vi "harp_connection_save_to_dev.vi"(0 "port in":refnum<visa-resource-name>) -> (4 "port out":refnum<visa-resource-name>, 8 "port closed":bool caption="Boolean", 15 "error out":errorcluster)   [LabVIEW 2010]
panel:
  in  "Visual Indicators:":enum8{"ON", "OFF"}(ring)
  in  "reset":bool caption="Boolean"
  in  "cancel":bool caption="Boolean"
  in  "LED State:":enum8{"ON", "OFF"}(ring)
  in  "Device State:":enum8{"Standby", "Active"}(ring)
  in  "read 5":bool
  in  "read 4":bool
  in  "read":bool
  in  "read 6":bool
  in  "read 7":bool
  in  "read 8":bool
  in  "read 3":bool
  in  "device":refnum<visa-resource-name>="COM5"
  in  "OK":bool caption="Boolean"
  # "Define the default state off the device."
  # "Configuration:"
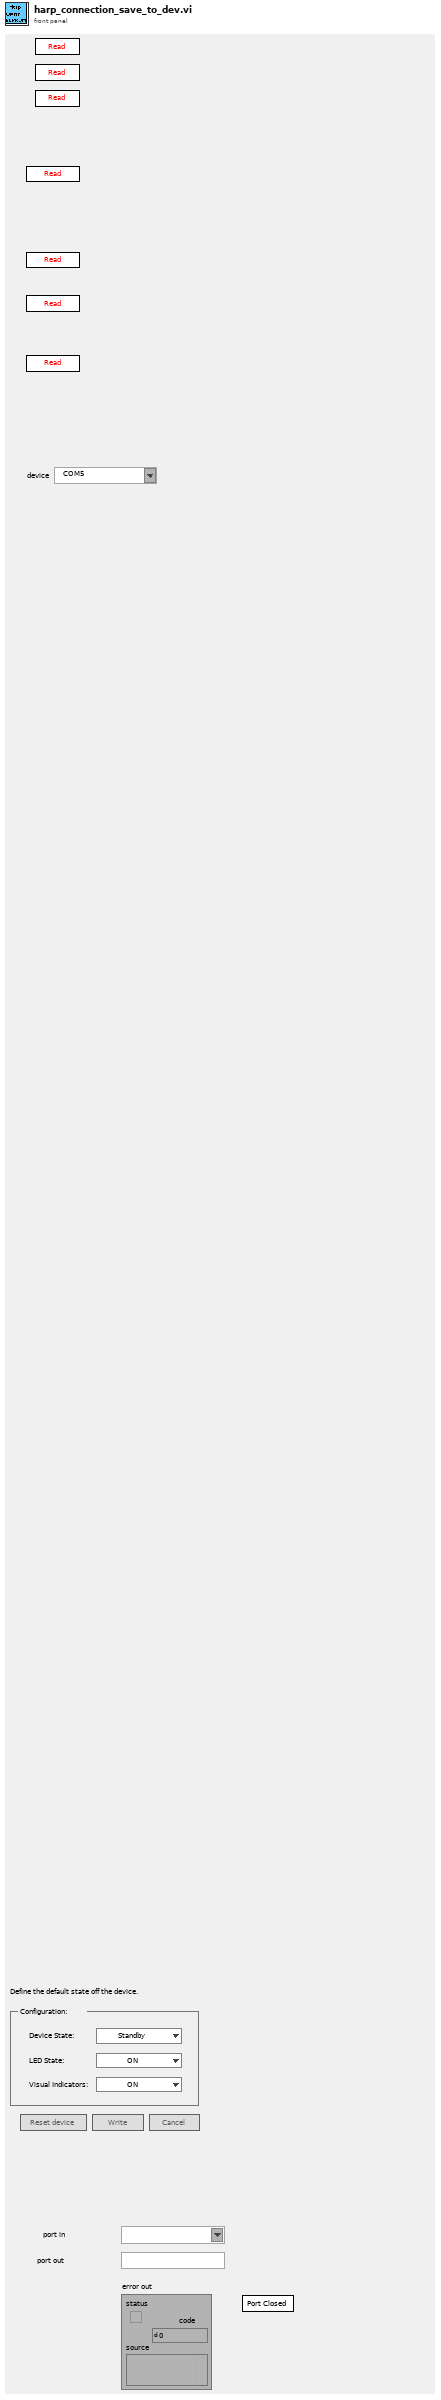
[diagram p1: front panel]
types:
  T1 = enum8{"Enabled", "Disabled", "Disabled and Grayed Out"}
  T2 = enum16{"Left Button", "Center Button", "Right Button", "Window Close"}
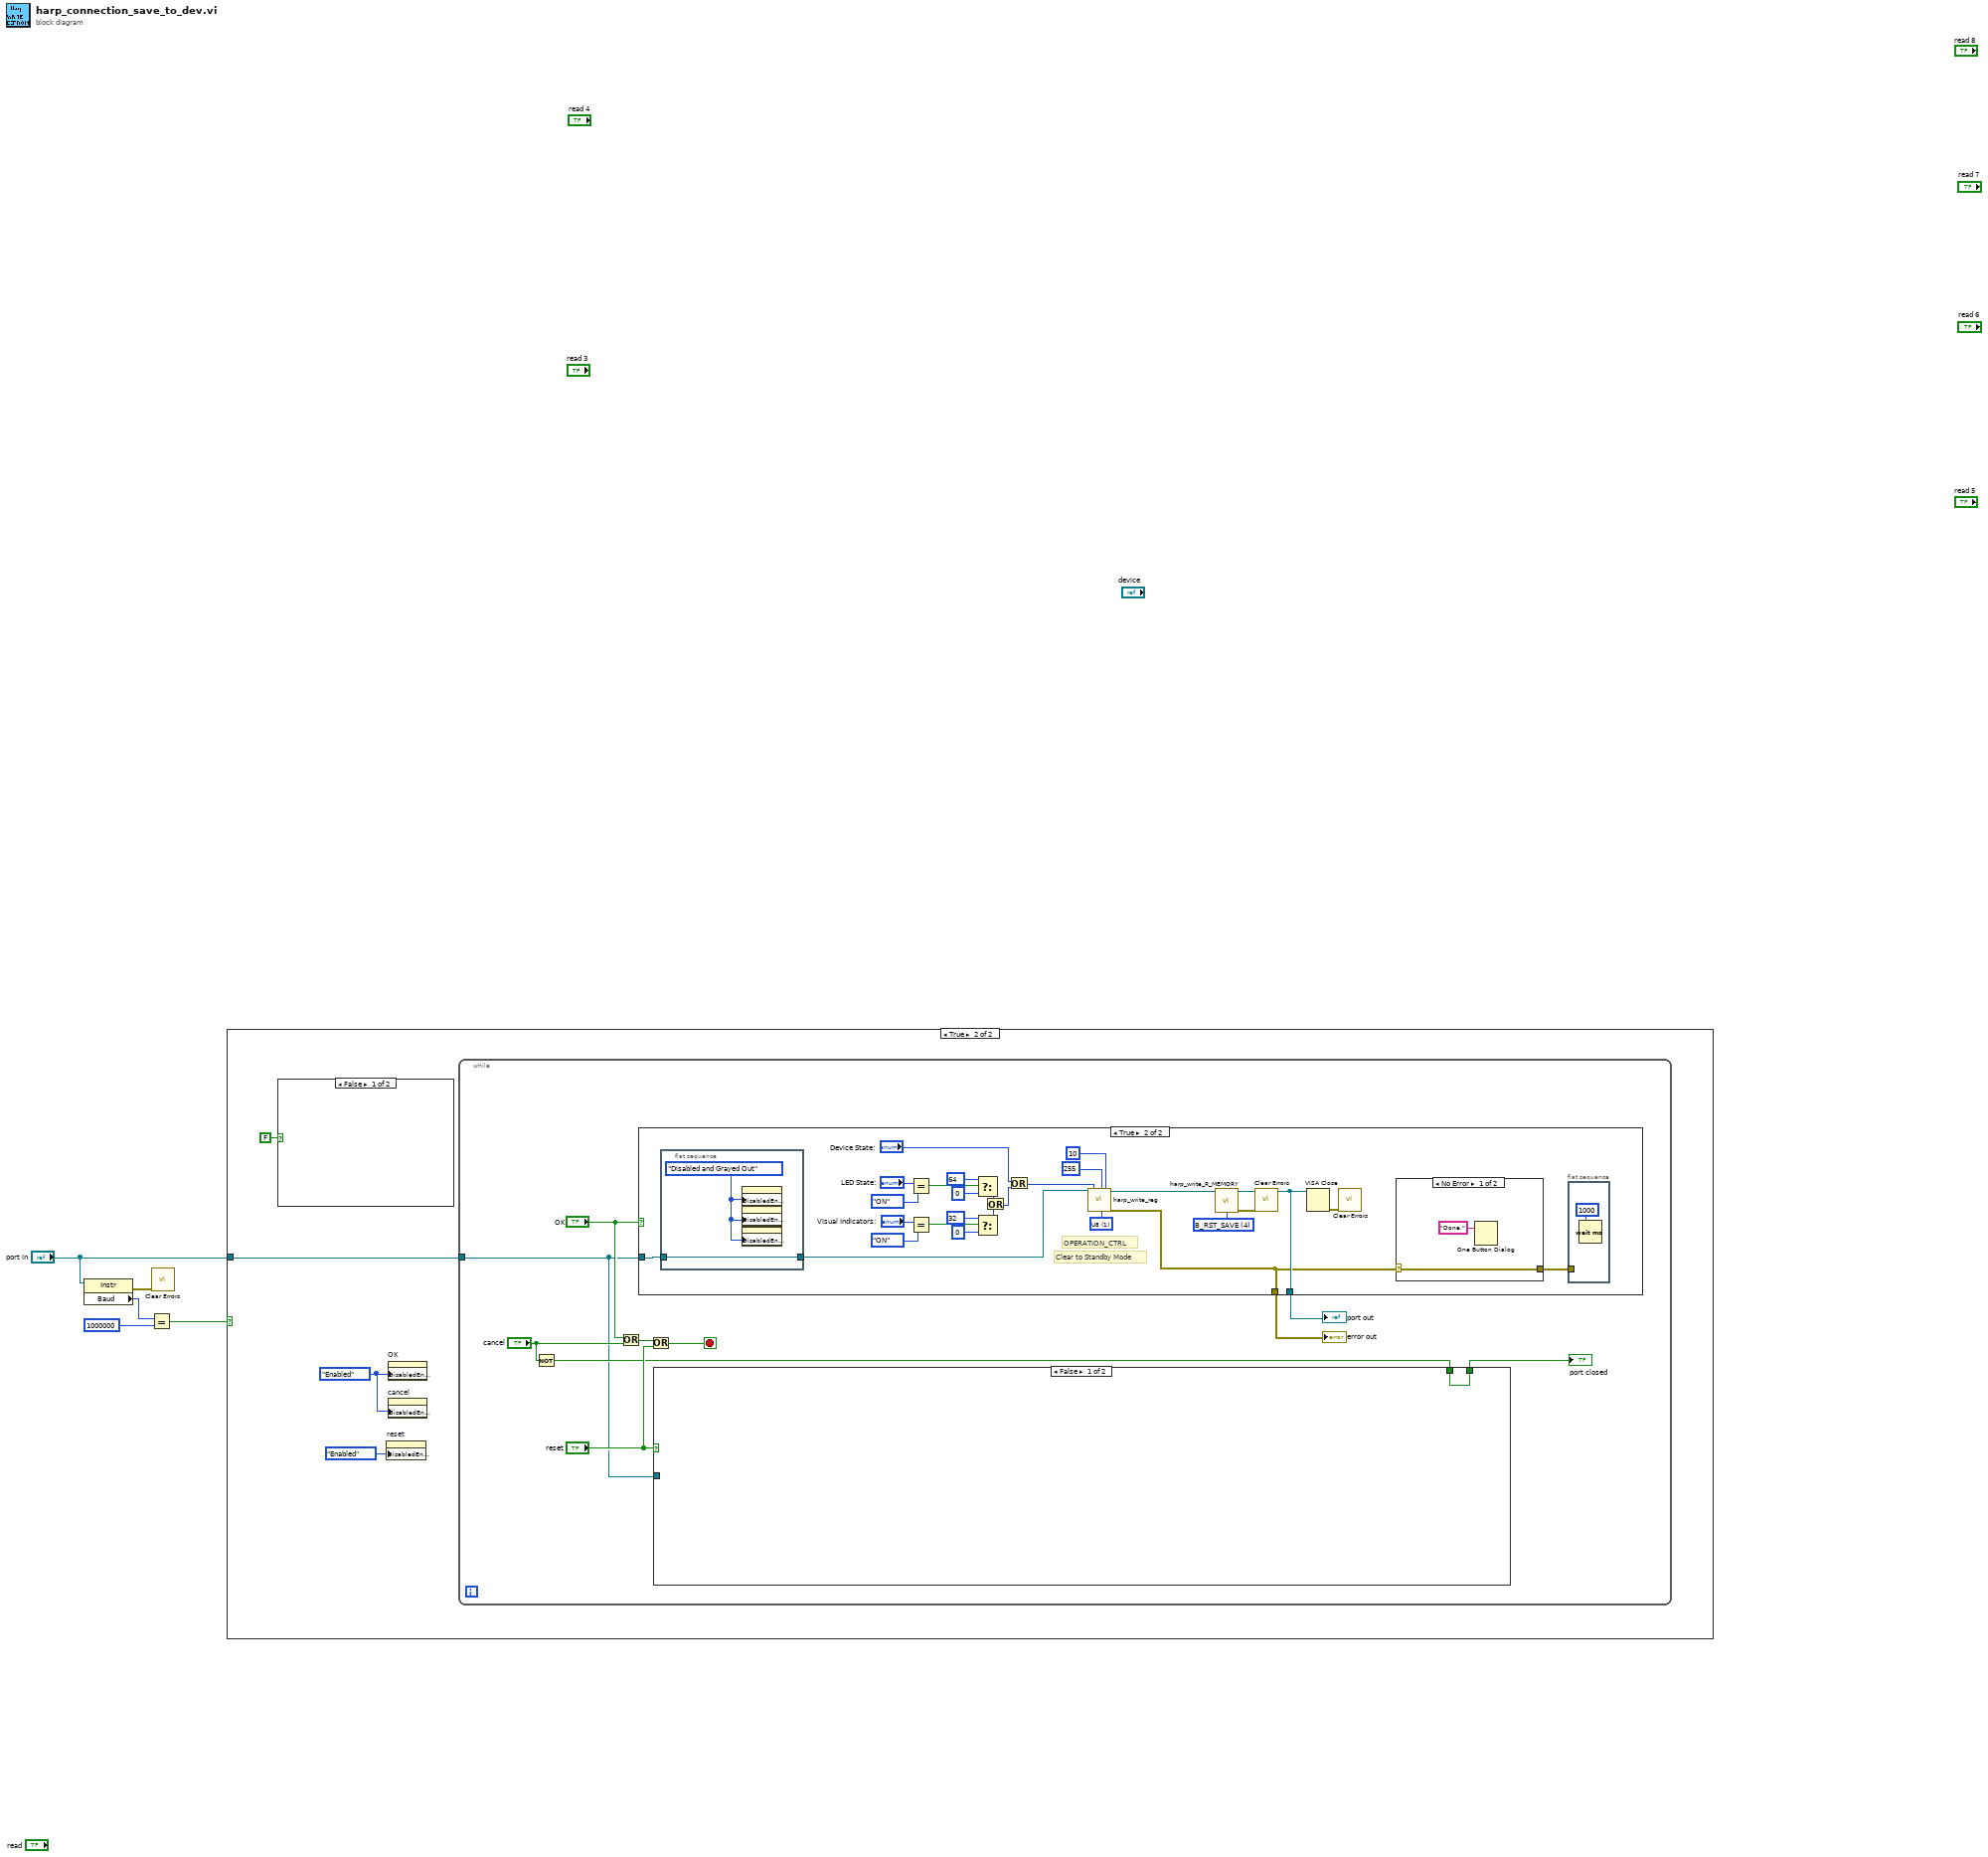
[diagram p0: block diagram]
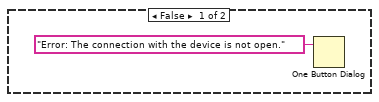
[diagram p2: hidden frame]
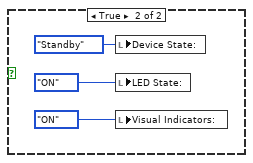
[diagram p3: hidden frame]
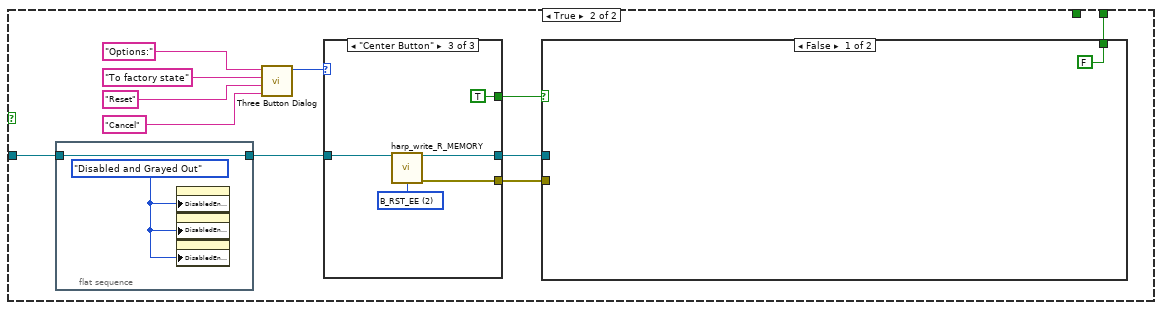
[diagram p4: hidden frame]
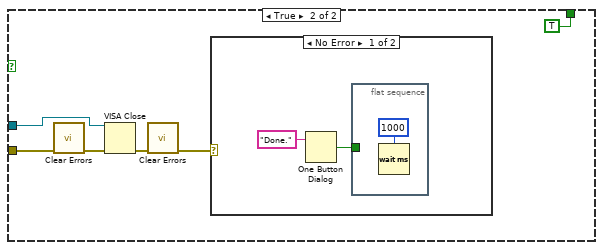
[diagram p5: hidden frame]
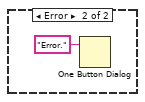
[diagram p6: hidden frame]
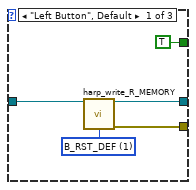
[diagram p7: hidden frame]
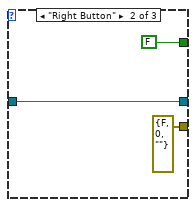
[diagram p8: hidden frame]
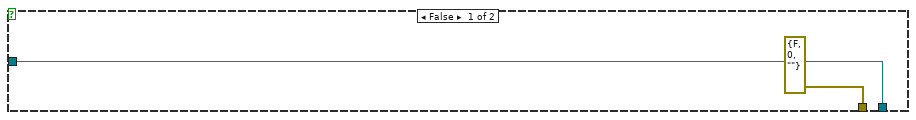
[diagram p9: hidden frame]
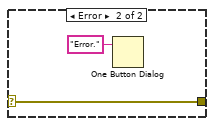
[diagram p10: hidden frame]
diagram:
  n1 = property class="Instr"(reference="port in") -> (error out=w3:errorcluster, "Baud"=w5:u32)  [unwired: 1 in, 1 out]
  n2 = Equal?(x=w5, y=u32 1000000) -> (x = y?=w1:bool)
  n3 = call <vilib>:"Clear Errors.vi"("error in (no error)"=w3) -> ()  [unwired: 6 in, 1 out]
  n4 = case shown="True" w1 {
    tunnel: "port in" -> [_ w7]
    frame False {
      n5 = One Button Dialog(message="Error: The connection with the device is not open.") -> ()  [unwired: 1 in, 1 out]
    }
    frame True {
      w10 = T1."Enabled" ("Disabled")
      n6 = case shown="False" FALSE {
        frame False {
        }
        frame True {
          n7 = local write "Device State:"(enum8{"Standby", "Active"}."Standby" ("Device Mode:")) -> ()
          n8 = local write "LED State:"(enum8{"ON", "OFF"}."ON" ("Indication LEDs:")) -> ()
          n9 = local write "Visual Indicators:"(enum8{"ON", "OFF"}."ON" ("Visual Indicators:")) -> ()
        }
      }
      n10 = property on="reset" class="Bool"("DisabledEnum"=T1."Enabled" ("Disabled")) -> ()  [unwired: 2 in, 2 out]
      n11 = property on="OK" class="Bool"("DisabledEnum"=w10) -> ()  [unwired: 2 in, 2 out]
      n12 = property on="cancel" class="Bool"("DisabledEnum"=w10) -> ()  [unwired: 2 in, 2 out]
      n13 = while {
        tunnel: w7 -> [w14]
        stop <- w19 stop-if-true
        n14 = Not(x="cancel") -> (.not. x?=w16:bool)
        n15 = Or(x="OK", y="cancel") -> (x .or. y?=w18:bool)
        n16 = case shown="True" "OK" {
          tunnel: w14 -> [w63 w78]
          tunnel: [w63 w75] -> w22
          tunnel: [errorcluster {"status"=FALSE, "code"=0, "source"=""} ("error out") w73] -> w23
          frame False {
          }
          frame True {
            w87 = u8 1 items=["U8"=1, "U16"=2, "U32"=4, "U64"=8, "I8"=129, "I16"=130, "I32"=132, "I64"=136, "FLOAT"=68, "BOOL"=17] ("type")
            w90 = u16 4 items=["B_RST_DEF"=1, "B_RST_EE"=2, "B_RST_SAVE"=4] ("Ring")
            # "Clear to Standby Mode"
            # "OPERATION_CTRL"
            n17 = flat-sequence {
              tunnel: w78 -> [w97]
              tunnel: [w97] -> w77
              frame #0 {
                w96 = T1."Disabled and Grayed Out" ("Disabled")
                n18 = property on="OK" class="Bool"("DisabledEnum"=w96) -> ()  [unwired: 2 in, 2 out]
                n19 = property on="cancel" class="Bool"("DisabledEnum"=w96) -> ()  [unwired: 2 in, 2 out]
                n20 = property on="reset" class="Bool"("DisabledEnum"=w96) -> ()  [unwired: 2 in, 2 out]
              }
            }
            n21 = Equal?(x="LED State:", y=enum8{"ON", "OFF"}."ON") -> (x = y?=w83:bool)
            n22 = Equal?(x="Visual Indicators:", y=enum8{"ON", "OFF"}."ON") -> (x = y?=w70:bool)
            n23 = Select(t=u8 64, s=w83, f=u8 0) -> (s? t:f=w65:u8)
            n24 = Select(t=u8 32, s=w70, f=u8 0) -> (s? t:f=w66:u8)
            n25 = Or(x=w65, y=w66) -> (x .or. y?=w64:u8)
            n26 = Or(x="Device State:", y=w64) -> (x .or. y?=w80:u8)
            n27 = call "harp_write_reg.vi"(0:"port"=w77, "8 bits"=w80, 10:"port"=u8 255 ("port"), "type"=w87, "reg. address"=u8 10) -> ("port out"=w79:refnum<visa-resource-name>, "error out"=w73:errorcluster)  [unwired: 12 in, 1 out]
            n28 = call "harp_write_R_MEMORY.vi"("port"=w79, "reset mode"=w90) -> ("port out"=w75:refnum<visa-resource-name>, "error out"=w72:errorcluster)  [unwired: 12 in]
            n29 = call <vilib>:"Clear Errors.vi"("error in (no error)"=w72) -> ()  [unwired: 6 in, 1 out]
            n30 = VISA Close(VISA resource name=w75) -> (error out=w74:errorcluster)  [unwired: 1 in]
            n31 = call <vilib>:"Clear Errors.vi"("error in (no error)"=w74) -> ()  [unwired: 6 in, 1 out]
            n32 = case shown="No Error" w73 {
              selector: w73 -> [w92 w94]
              tunnel: [w92 w94] -> w76
              frame No Error {
                n33 = One Button Dialog(message="Done.") -> ()  [unwired: 1 in, 1 out]
              }
              frame Error {
                n34 = One Button Dialog(message="Error.") -> ()  [unwired: 1 in, 1 out]
              }
            }
            n35 = flat-sequence {
              tunnel: w76 -> [_]
              frame #0 {
                n36 = Wait (ms)(milliseconds to wait=u32 1000) -> ()  [unwired: 1 out]
              }
            }
          }
        }
        "port out" <- w22
        "error out" <- w23
        n37 = Or(x=w18, y="reset") -> (x .or. y?=w19:bool)
        n38 = case shown="False" "reset" {
          tunnel: w14 -> [_ w28]
          tunnel: [w24 w25] -> w15
          tunnel: w16 -> [w24 _]
          frame False {
          }
          frame True {
            n39 = flat-sequence {
              tunnel: w28 -> [w37]
              tunnel: [w37] -> w27
              frame #0 {
                w36 = T1."Disabled and Grayed Out" ("Disabled")
                n40 = property on="reset" class="Bool"("DisabledEnum"=w36) -> ()  [unwired: 2 in, 2 out]
                n41 = property on="OK" class="Bool"("DisabledEnum"=w36) -> ()  [unwired: 2 in, 2 out]
                n42 = property on="cancel" class="Bool"("DisabledEnum"=w36) -> ()  [unwired: 2 in, 2 out]
              }
            }
            n43 = call <vilib>:"Three Button Dialog.vi"("Right Button Text (\"Cancel\")"="Cancel" ("Center Button Text (\"No\")"), "Center Button Text (\"No\")"="Reset" ("Center Button Text (\"No\")"), "Left Button Text (\"Yes\")"="To factory state" ("Left Button Text (\"Yes\")"), "message"="Options:") -> ("Which Button?"=w31:T2)  [unwired: 7 in]
            n44 = case shown="\"Center Button\"" w31 {
              tunnel: w27 -> [w52 w54 w60]
              tunnel: [w51 errorcluster {"status"=FALSE, "code"=0, "source"=""} ("error out") w59] -> w30
              tunnel: [TRUE FALSE TRUE] -> w29
              tunnel: [w49 w54 w57] -> w26
              frame "Left Button", Default {
                w53 = u16 1 items=["B_RST_DEF"=1, "B_RST_EE"=2, "B_RST_SAVE"=4] ("Ring")
                n45 = call "harp_write_R_MEMORY.vi"("port"=w52, "reset mode"=w53) -> ("port out"=w49:refnum<visa-resource-name>, "error out"=w51:errorcluster)  [unwired: 12 in]
              }
              frame "Right Button" {
              }
              frame "Center Button" {
                w61 = u16 2 items=["B_RST_DEF"=1, "B_RST_EE"=2, "B_RST_SAVE"=4] ("Ring")
                n46 = call "harp_write_R_MEMORY.vi"("port"=w60, "reset mode"=w61) -> ("port out"=w57:refnum<visa-resource-name>, "error out"=w59:errorcluster)  [unwired: 12 in]
              }
            }
            n47 = case shown="False" w29 {
              tunnel: w30 -> [_ w43]
              tunnel: w26 -> [_ w41]
              tunnel: [FALSE TRUE] -> w25
              frame False {
              }
              frame True {
                n48 = call <vilib>:"Clear Errors.vi"("error in (no error)"=w43) -> ("error out"=w40:errorcluster)  [unwired: 6 in]
                n49 = VISA Close(VISA resource name=w41, error in (no error)=w40) -> (error out=w44:errorcluster)
                n50 = call <vilib>:"Clear Errors.vi"("error in (no error)"=w44) -> ("error out"=w42:errorcluster)  [unwired: 6 in]
                n51 = case shown="No Error" w42 {
                  frame No Error {
                    n52 = One Button Dialog(message="Done.") -> (true=w45:bool)  [unwired: 1 in]
                    n53 = flat-sequence {
                      tunnel: w45 -> [_]
                      frame #0 {
                        n54 = Wait (ms)(milliseconds to wait=u32 1000) -> ()  [unwired: 1 out]
                      }
                    }
                  }
                  frame Error {
                    n55 = One Button Dialog(message="Error.") -> ()  [unwired: 1 in, 1 out]
                  }
                }
              }
            }
          }
        }
        "port closed" <- w15
      }
    }
  }
